vi "multi button dialog.vi"(8 "error in (no error)":errorcluster) -> (0 "error out":errorcluster)   [LabVIEW 2013]
uses:
  Dialog Icon names enum.ctl
  Dialog Icon control.ctl
  <vilib>/Utility/miscctls.llb/LVPointTypeDef.ctl
panel:
  in  "Button 1":bool
  in  "Button 2":bool
  out "Message":string
  out "Dialog Icon":T1
  in  "Timeout sec (-1)":dbl
  in  "Settings":cluster{"Panel Color":u32, "Icon":T2}
  # "Title('')\nState (Modal)\nMessage ('')\nColor (system panel\nButtons[ ]\nFont ref?(default)\nicon(None)\nsize\nmonitor"
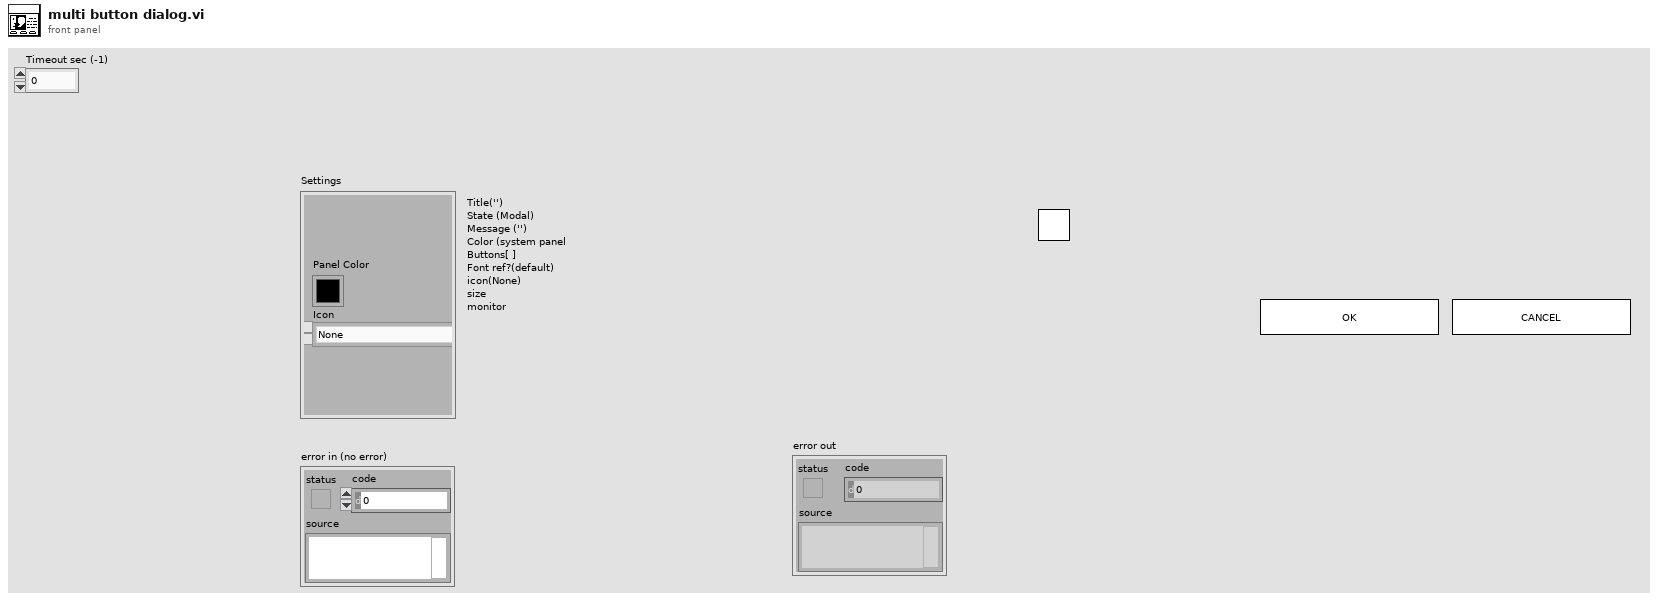
[diagram p1: front panel]
types:
  T1 = typedef "Dialog Icon control.ctl" = u16
  T2 = typedef "Dialog Icon names enum.ctl" = enum16{"None", "Exclamation", "Question", "Error", "Information"}
  T3 = typedef "LVPointTypeDef.ctl" = cluster{"Horizontal":i16, "Vertical":i16}
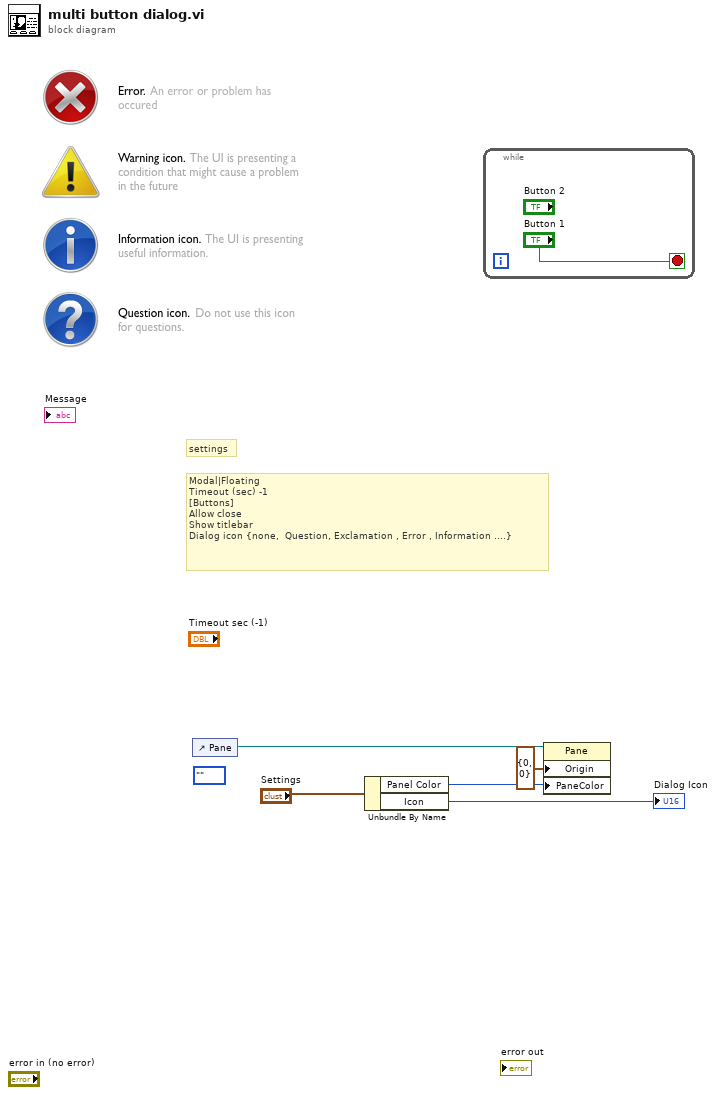
[diagram p0: block diagram]
diagram:
  (unwired) enum16{""}.""
  # "settings"
  # "Modal|Floating\nTimeout (sec) -1\n[Buttons]\nAllow close\nShow titlebar\nDialog icon {none,  Question, Exclamation , Error , Information ....}"
  n1 = control-ref of="Pane"() -> (w4:refnum<vi>)
  n2 = Unbundle By Name("Settings") -> ("Panel Color"=w2:u32, "Icon"=→"Dialog Icon":T2)
  n3 = while {
    stop <- "Button 1" stop-if-true
  }
  n4 = property class="Pane"(reference=w4, "Origin"=T3 {"Horizontal"=0, "Vertical"=0}, "PaneColor"=w2) -> ()  [unwired: 1 in, 2 out]
